vi "SwerveJoystickStrafeScaling.vi"(4 "Raw Y Joystick":dbl, 5 "Raw X Joystick":dbl, 6 "Strafe Scaling":dbl(slide)=2.0 min=1.0 max=4.0 scale=1.0..4.0, 7 "Strafe Deadband":dbl(slide)=0.05 min=0.0 max=0.4 scale=0.0..0.4) -> (0 "Scaled Y Joystick":dbl, 1 "Scaled X Joystick":dbl, 3 "Out of Deadband":bool)   [LabVIEW 2019]
doc: "Applies a deadband and nonlinear scaling to the strafe axes of a swerve drive."
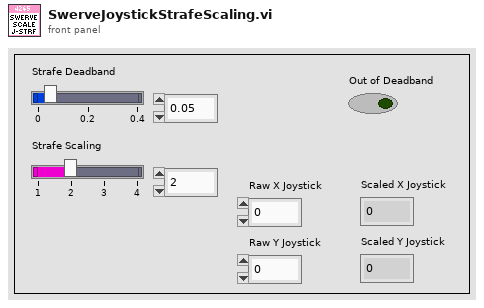
[diagram p1: front panel]
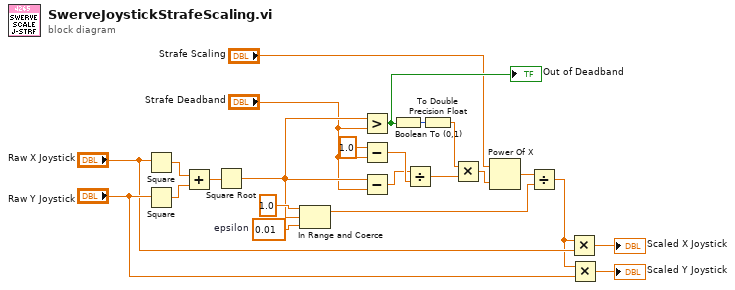
[diagram p0: block diagram]
diagram:
  w13 = 0.01  # epsilon
  n1 = Square(x="Raw X Joystick") -> (x^2=w10:dbl)
  n2 = Square(x="Raw Y Joystick") -> (x^2=w9:dbl)
  n3 = Add(x=w10, y=w9) -> (x+y=w11:dbl)
  n4 = Square Root(x=w11) -> (sqrt(x)=w14:dbl)
  n5 = In Range and Coerce(upper limit=1.0, x=w14, lower limit=w13) -> (coerced(x)=w12:dbl)  [unwired: 1 out]
  n6 = Greater?(x=w14, y="Strafe Deadband") -> (0:w21:bool)
  "Out of Deadband" <- w21
  n7 = Subtract(x=1.0, y="Strafe Deadband") -> (x-y=w7:dbl)
  n8 = Subtract(x=w14, y="Strafe Deadband") -> (x-y=w5:dbl)
  n9 = Boolean To (0,1)(Boolean=w21) -> (0, 1=w3:i16)
  n10 = Divide(x=w5, y=w7) -> (x/y=w8:dbl)
  n11 = To Double Precision Float(number=w3) -> (double precision float=w4:dbl)
  n12 = Multiply(x=w4, y=w8) -> (x*y=w22:dbl)
  n13 = Power Of X(1:w22, 2:"Strafe Scaling") -> (0:w23:dbl)
  n14 = Divide(x=w23, y=w12) -> (x/y=w16:dbl)
  n15 = Multiply(x=w16, y="Raw X Joystick") -> (x*y=→"Scaled X Joystick":dbl)
  n16 = Multiply(x=w16, y="Raw Y Joystick") -> (x*y=→"Scaled Y Joystick":dbl)
